vi "模拟输出_软件按需单点_电流.vi"() -> ()   [LabVIEW 2013]
doc: "This example demonstrates how to output a single voltage."
uses:
  <userlib>/ArtDAQ/_SubVI/ArtDAQ_CreateAOCurrentChan.vi
  <userlib>/ArtDAQ/_SubVI/ArtDAQ_Write Analog DBL NChan 1Samp.vi
panel:
  in  "通道1(A)":dbl=0.005 format="%#_13g"
  in  "通道0 (A)":dbl=0.01 format="%#_13g"
  in  "Stop":bool
  in  "最大值(A)":dbl=0.02
  in  "最小值(A)":dbl=-0.02
  in  "物理通道":string="Dev1/ao0:1"
  out "错误输出":errorcluster
  # "通道属性"
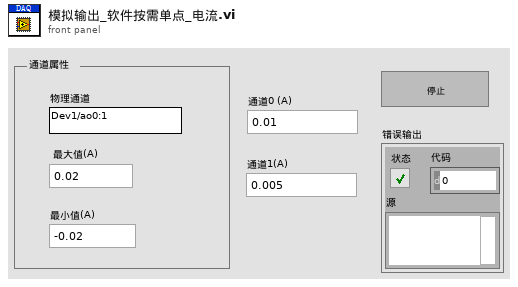
[diagram p1: front panel]
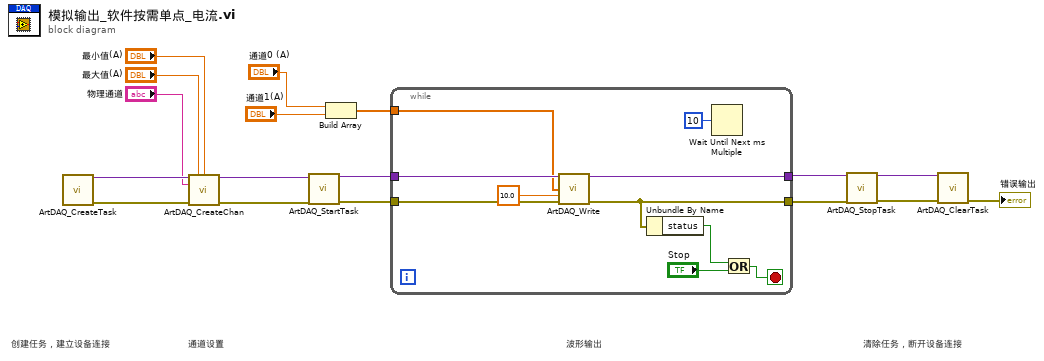
[diagram p0: block diagram]
diagram:
  # "清除任务，断开设备连接"
  # "波形输出"
  # "通道设置"
  # "创建任务，建立设备连接"
  n1 = call <userlib>:"ArtDAQ_CreateTask.vi"() -> ("任务句柄"=w17:variant, "错误输出"=w16:errorcluster)  [unwired: 14 in]
  n2 = call-poly <userlib>:"ArtDAQ_CreateChan.vi"("任务句柄"=w17, "最大值"="最大值(A)", "最小值"="最小值(A)", "物理通道"="物理通道", "错误输入"=w16) -> ("任务句柄"=w9:variant, "错误输出"=w8:errorcluster)  [unwired: 9 in]
  n3 = call <userlib>:"ArtDAQ_StartTask.vi"("任务句柄"=w9, "错误输入"=w8) -> ("任务句柄"=w7:variant, "错误输出"=w6:errorcluster)  [unwired: 12 in]
  n4 = Build Array("通道0 (A)", "通道1(A)") -> (w1:dbl[])
  n5 = while {
    tunnel: w7 -> [w26]
    tunnel: w6 -> [w25]
    tunnel: [w24] -> w5
    tunnel: [w19] -> w4
    tunnel: w1 -> [w18]
    stop <- w20 stop-if-true
    n6 = call-poly <userlib>:"ArtDAQ_Write.vi"("任务句柄"=w26, "数据"=w18, "超时s"=10.0 ("Timeout"), "错误输入"=w25) -> ("任务句柄"=w24:variant, "错误输出"=w19:errorcluster)  [unwired: 10 in]
    n7 = Unbundle By Name(w19) -> ("status"=w21:bool)
    n8 = Wait Until Next ms Multiple(millisecond multiple=u32 10 ("毫秒倍数")) -> ()  [unwired: 1 out]
    n9 = Or(x=w21, y="Stop") -> (x .or. y?=w20:bool)
  }
  n10 = call <userlib>:"ArtDAQ_StopTask.vi"("任务句柄"=w5, "错误输入"=w4) -> ("任务句柄"=w15:variant, "错误输出"=w14:errorcluster)  [unwired: 12 in]
  n11 = call <userlib>:"ArtDAQ_ClearTask.vi"("任务句柄"=w15, "错误输入"=w14) -> ("错误输出"=→"错误输出":errorcluster)  [unwired: 13 in]
